vi "get_LV_version.vi"(8 "error in (no error)":errorcluster, 9 "string in":string) -> (0 "error out":errorcluster, 1 "edited string out":string)   [LabVIEW 2010, in "ErrorController.lvclass"]
uses:
  ErrorController.lvclass
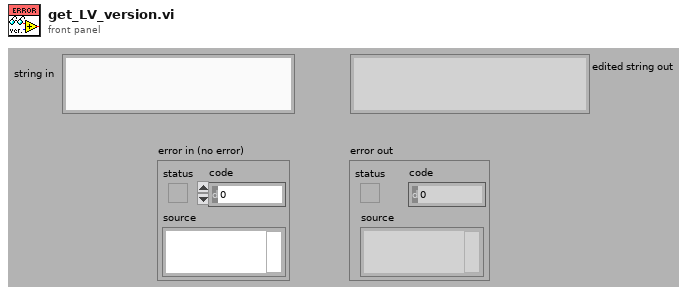
[diagram p1: front panel]
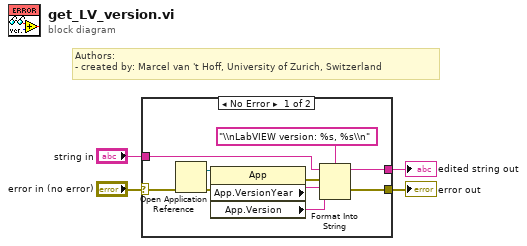
[diagram p0: block diagram]
diagram:
  # "Authors: \n- created by: Marcel van 't Hoff, University of Zurich, Switzerland"
  n1 = case shown="No Error" "error in (no error)" {
    selector: "error in (no error)" -> [w6 w15]
    tunnel: [w7 w15] -> w3
    tunnel: "string in" -> [w12 _]
    tunnel: [w8 _] -> w1
    frame No Error {
      n2 = Open Application Reference(8:w6) -> (0:w13:errorcluster, 3:w14:refnum<vi>)  [unwired: 3 in]
      n3 = property class="App"(reference=w14, error in=w13) -> (error out=w10:errorcluster, "App.VersionYear"=w9:string, "App.Version"=w5:string)  [unwired: 1 out]
      n4 = Format Into String(format string="\\nLabVIEW version: %s, %s\\n", initial string=w12, error in=w10, w9, w5) -> (resulting string=w8:string, error out=w7:errorcluster)
    }
    frame Error {
    }
  }
  "error out" <- w3
  "edited string out" <- w1
